vi "Write ChannelData.vi"(8 "error in (no error)":errorcluster, 10 "Channel.lvlib:ChannelData.lvclass":refnum<class "ChannelData.lvclass">, 11 "Channel in":refnum<class "Channel.lvclass">) -> (0 "error out":errorcluster, 3 "Channel out":refnum<class "Channel.lvclass">)   [LabVIEW 2015, in "Channel.lvlib" / "Channel.lvclass"]
uses:
  Channel.lvclass
  ChannelData.lvclass
  Channel.lvclass/Channel.ctl
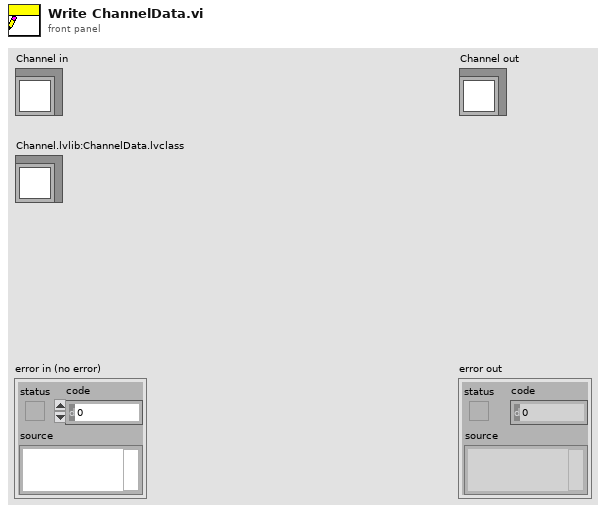
[diagram p1: front panel]
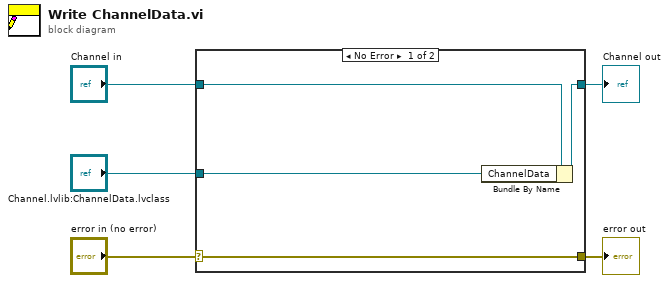
[diagram p0: block diagram]
diagram:
  n1 = case shown="No Error" "error in (no error)" {
    selector: "error in (no error)" -> [w9 w10]
    tunnel: [w9 w10] -> w4
    tunnel: [w7 w11] -> w2
    tunnel: "Channel in" -> [w8 w11]
    tunnel: "Channel.lvlib:ChannelData.lvclass" -> [w6 _]
    frame No Error {
      n2 = Bundle By Name(cluster=w8, "ChannelData"=w6) -> (w7:refnum<class "Channel.lvclass">)
    }
    frame Error {
    }
  }
  "error out" <- w4
  "Channel out" <- w2
